vi "Request voltage CH2 (SubVI).vi"() -> (3 "Request voltage CH2 / Y":string)   [LabVIEW 2018]
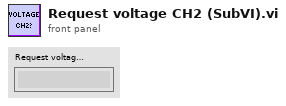
[diagram p1: front panel]
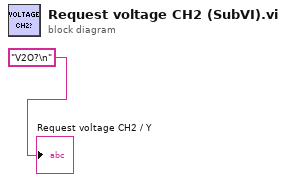
[diagram p0: block diagram]
diagram:
  "Request voltage CH2 / Y" <- "V2O?\n" ("format string")
